vi "testGetServerNotifier(cmd).vi"(8 "error in (no error)":errorcluster) -> (0 "error out":errorcluster)   [LabVIEW 2018]
doc: "Test the getServerNotifier.vi."
uses:
  src/TcpServer/TcpServer.lvclass
  src/TcpServer/TcpServer.lvclass/TcpServer.ctl
  src/TcpServerCmd/TcpServerCmd.lvclass
  home/pcortes/github/ts_labview_tcp_json/src/TcpServerBase/TcpServerBase.lvclass
  <vilib>/addons/_JKI Toolkits/Caraya/classes/Assert/Assert Equal Type_Variant.vi
  <vilib>/addons/_JKI Toolkits/Caraya/classes/Test/Test.lvclass
  <vilib>/addons/_JKI Toolkits/Caraya/classes/Assert/Assert.lvclass
  src/TcpServerBase/TcpServerBase.lvclass
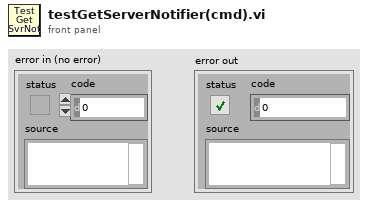
[diagram p1: front panel]
types:
  T1 = cluster{"connectionStatus":bool, "errorSource":string}
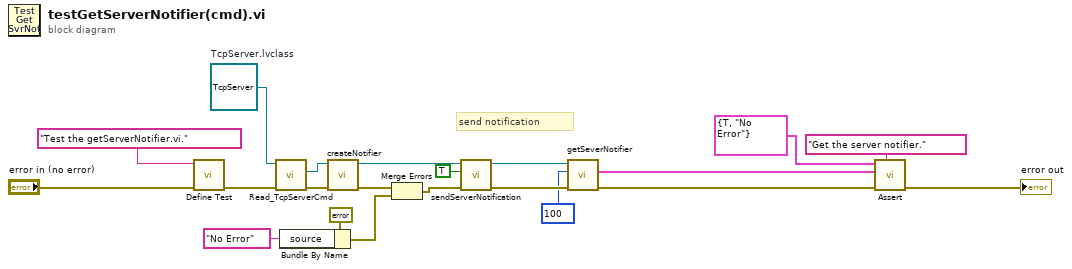
[diagram p0: block diagram]
diagram:
  w9 = refnum<class "TcpServer.lvclass"> refnum  # TcpServer.lvclass
  # "send notification"
  n1 = call <vilib>:"Define Test.vi"("error in (no error)"="error in (no error)", "Label (VI Title)"="Test the getServerNotifier.vi.") -> ("error out"=w6:errorcluster)  [unwired: 9 in]
  n2 = call "Read_TcpServerCmd.vi"("error in (no error)"=w6, "TcpServer in"=w9) -> ("error out"=w7:errorcluster, "TcpServerCmd.lvclass"=w8:refnum<class "TcpServerCmd.lvclass">)  [unwired: 7 in, 1 out]
  n3 = Bundle By Name(cluster=errorcluster {"status"=FALSE, "code"=0, "source"=""} ("error in (no error)"), "source"="No Error") -> (w12:errorcluster)
  n4 = call "createNotifier.vi"("error in (no error)"=w7, "tcpServerBase in"=w8) -> ("error out"=w11:errorcluster, "tcpServerBase out"=w18:refnum<class "TcpServerCmd.lvclass">)  [unwired: 8 in]
  n5 = Merge Errors(w11, w12) -> (w13:errorcluster)
  n6 = call "sendServerNotification.vi"("error in (no error)"=w13, "serverStatus"=TRUE, "TcpServerBase in"=w18) -> ("error out"=w4:errorcluster, "TcpServerBase out"=w5:refnum<class "TcpServerCmd.lvclass">)  [unwired: 7 in]
  n7 = call "getSeverNotifier.vi"("error in (no error)"=w4, "Timeout Notifier"=100, "TcpServerBase in"=w5) -> ("error out"=w1:errorcluster, "connStatusCluster"=w2:T1)  [unwired: 5 in, 2 out]
  n8 = call-poly <vilib>:"Assert.vi"("Label"="Get the server notifier.", "error in (no error)"=w1, "Y"=w2, "X"=T1 {"connectionStatus"=TRUE, "errorSource"="No Error"} ("notification")) -> ("error out"=→"error out":errorcluster)  [unwired: 7 in]
